vi "workbook add chartsheet lv.vi"(8 "error in (no error)":errorcluster, 10 "sheetname":string, 11 "workbook":u32) -> (0 "error out":errorcluster, 3 "function return":u32)   [LabVIEW 2015, in "xlsxwriter.lvlib"]
doc: "lxw_chartsheet workbook_add_chartsheet_lv(lxw_workbook workbook, const char *sheetname);"
uses:
  xlsxwriter.lvlib
  xlsxwriter.dll
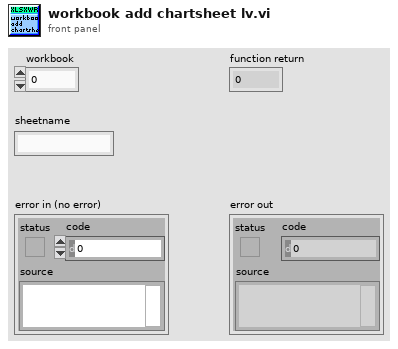
[diagram p1: front panel]
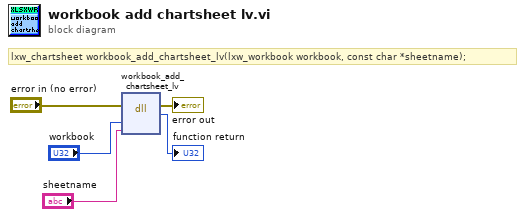
[diagram p0: block diagram]
diagram:
  # "lxw_chartsheet workbook_add_chartsheet_lv(lxw_workbook workbook, const char *sheetname);"
  n1 = dll-call lib="C:/Users/WDAGUtilityAccount/Desktop/lv_vis_added_cell/xlsxwriter.*" fn="workbook_add_chartsheet_lv"(error in="error in (no error)", "workbook"="workbook", "sheetname"="sheetname") -> (error out=→"error out":errorcluster, →"function return":u32)  [unwired: 4 in, 1 out]
